vi "Post-Build Action.vi"(5 "Files Generated by Build":path[](array[path]), 6 "Top Level/Always Included VIs":path[](array[path]), 7 "Destination Path":path, 8 "error in (no error)":errorcluster, 9 "Target Name":string, 10 "Build Specification Name":string, 11 "Project Path":path) -> (0 "error out":errorcluster)   [LabVIEW 2020]
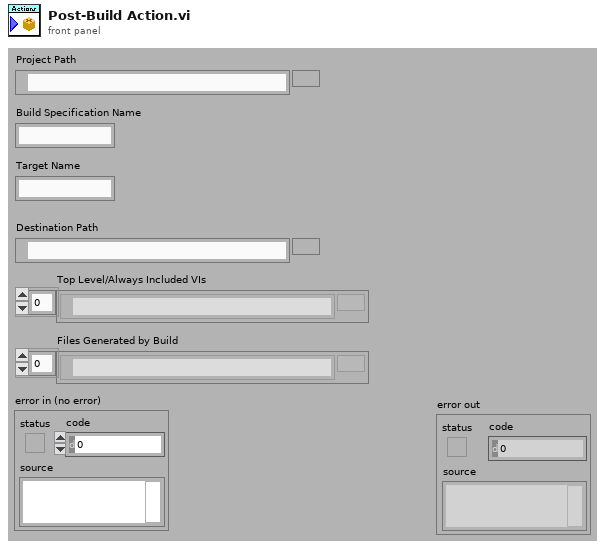
[diagram p1: front panel]
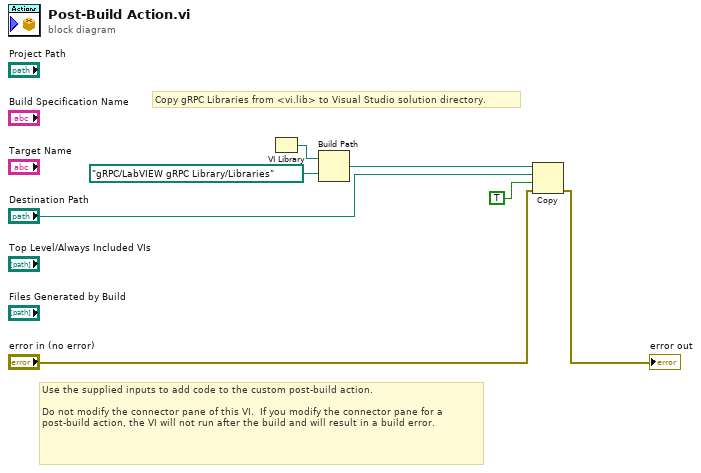
[diagram p0: block diagram]
diagram:
  # "Copy gRPC Libraries from <vi.lib> to Visual Studio solution directory."
  # "Use the supplied inputs to add code to the custom post-build action.\n\nDo not modify the connector pane of this VI.  If you modify the connector pane for a post-build action, the VI will not run after the build and will result in a build error."
  n1 = VI Library() -> (path=w7:path)
  n2 = Build Path(base path=w7, name or relative path=path "gRPC/LabVIEW gRPC Library/Libraries" ("path")) -> (appended path=w5:path)
  n3 = Copy(8:"error in (no error)", 9:TRUE ("overwrite (F)"), 10:"Destination Path", 11:w5) -> (0:→"error out":errorcluster)  [unwired: 1 in, 2 out]
